vi "Boolean Output Item Resize.vi"(8 "error in (no error)":errorcluster, 9 "NewBnds":T2, 10 "Bool UI Elements":T1) -> (0 "error out":errorcluster)   [LabVIEW 2015, in "OutputUI.lvclass"]
uses:
  OutputUI.lvclass
  <vilib>/Utility/miscctls.llb/LVRectTypeDef.ctl
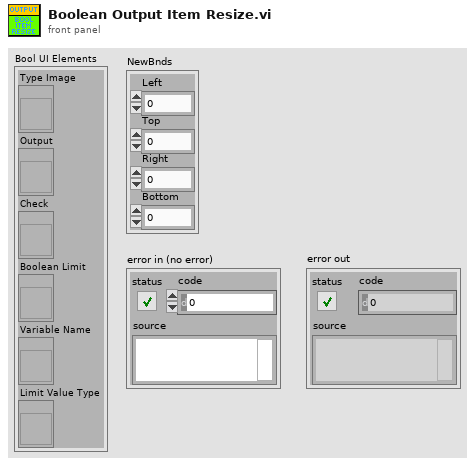
[diagram p1: front panel]
types:
  T1 = cluster{"Type Image":refnum<vi>, "Output":refnum<vi>, "Check":refnum<vi>, "Boolean Limit":refnum<vi>, "Variable Name":refnum<vi>, "Limit Value Type":refnum<vi>}
  T2 = typedef "LVRectTypeDef.ctl" = cluster{"Left":i16, "Top":i16, "Right":i16, "Bottom":i16}
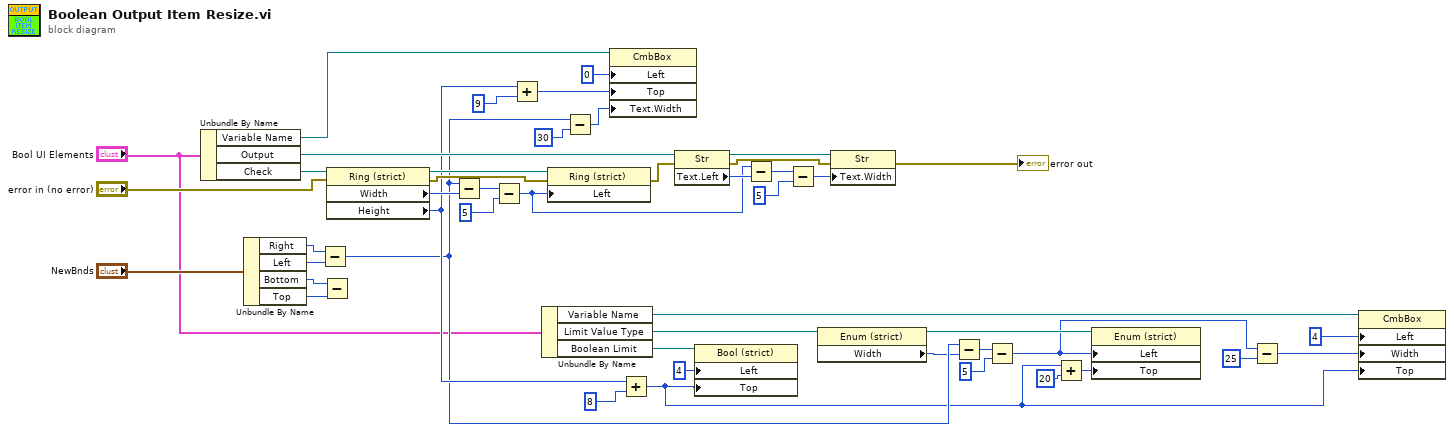
[diagram p0: block diagram]
diagram:
  n1 = Unbundle By Name("Bool UI Elements") -> ("Variable Name"=w25:refnum<vi>, "Output"=w39:refnum<vi>, "Check"=w47:refnum<vi>)
  n2 = Unbundle By Name("NewBnds") -> ("Right"=w44:i16, "Left"=w45:i16, "Bottom"=w43:i16, "Top"=w42:i16)
  n3 = Subtract(x=w44, y=w45) -> (x-y=w19:i16)
  n4 = Subtract(x=w43, y=w42) -> ()  [unwired: 1 out]
  n5 = property class="Ring (strict)"(reference=w47, error in="error in (no error)") -> (reference out=w41:refnum<vi>, error out=w28:errorcluster, "Width"=w40:u32, "Height"=w21:u32)
  n6 = Subtract(x=w19, y=w40) -> (x-y=w36:u32)
  n7 = Subtract(x=w36, y=5) -> (x-y=w34:u32)
  n8 = Add(x=w21, y=9) -> (x+y=w22:u32)
  n9 = Unbundle By Name("Bool UI Elements") -> ("Variable Name"=w10:refnum<vi>, "Limit Value Type"=w13:refnum<vi>, "Boolean Limit"=w16:refnum<vi>)
  n10 = property class="Ring (strict)"(reference=w41, error in=w28, "Left"=w34) -> (error out=w27:errorcluster)  [unwired: 1 out]
  n11 = Subtract(x=w19, y=30) -> (x-y=w20:i32)
  n12 = property class="CmbBox"(reference=w25, "Left"=0 ("Position:Left"), "Top"=w22, "Text.Width"=w20) -> ()  [unwired: 1 in, 2 out]
  n13 = Add(x=w21, y=8) -> (x+y=w6:u32)
  n14 = property class="Str"(reference=w39, error in=w27) -> (reference out=w38:refnum<vi>, error out=w26:errorcluster, "Text.Left"=w37:i32)
  n15 = property class="Bool (strict)"(reference=w16, "Left"=4 ("Position:Left"), "Top"=w6) -> ()  [unwired: 1 in, 2 out]
  n16 = Subtract(x=w34, y=w37) -> (x-y=w33:u32)
  n17 = Subtract(x=w33, y=u32 5) -> (x-y=w32:u32)
  n18 = property class="Enum (strict)"(reference=w13) -> (reference out=w12:refnum<vi>, "Width"=w11:u32)  [unwired: 1 in, 1 out]
  n19 = property class="Str"(reference=w38, error in=w26, "Text.Width"=w32) -> (error out=→"error out":errorcluster)  [unwired: 1 out]
  n20 = Subtract(x=w19, y=w11) -> (x-y=w3:u32)
  n21 = Subtract(x=w3, y=u32 5) -> (x-y=w1:u32)
  n22 = Add(x=w6, y=u32 20) -> (x+y=w5:u32)
  n23 = property class="Enum (strict)"(reference=w12, "Left"=w1, "Top"=w5) -> ()  [unwired: 1 in, 2 out]
  n24 = Subtract(x=w1, y=u32 25) -> (x-y=w7:u32)
  n25 = property class="CmbBox"(reference=w10, "Left"=4 ("Position:Left"), "Width"=w7, "Top"=w6) -> ()  [unwired: 1 in, 2 out]
